vi "LV86_Histograph.vi"(3 "Image":T1 {"Dialogs" format="%.0b"}) -> (0 "Histogram":i32[](graph), 1 "Image Out":T1 {"Dialogs" format="%.0b"})   [LabVIEW 2024]
doc: "This VI automatically thresholds an image (clustering method). Pixels within the determined range maintain their original value, while pixels outside this range are given the value 0. (Does not work with color images)"
uses:
  <userlib>/ImageProcessing/QTLIB_2595_LV86/QT_Image.ctl
  <vilib>/Analysis/NI_AALPro.lvlib
panel:
  # "This VI automatically thresholds an image(clustering method).\nPixels within the determined range  maintain their original value, while pixels outside this range are given the value 0.   (Does not work with color images)"
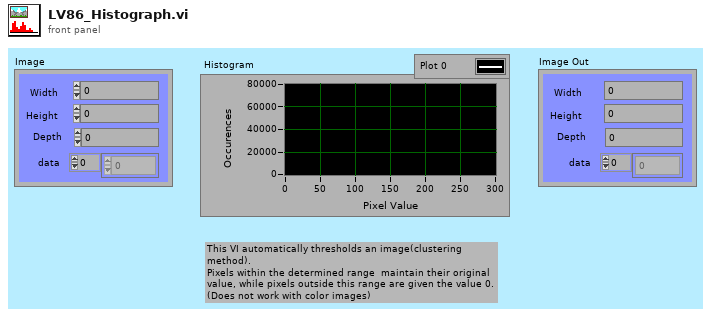
[diagram p1: front panel]
types:
  T1 = typedef "QT_Image.ctl" = cluster{"Width":i32, "Height":i32, "Depth":i32, "data":u8[], "Compressed data":u8[], "Color table":u32[], "Duration":i32, "Options":i32, "Timestamp":i32, "ID":i32, "Reserved":i32, "Dialogs":u32}
  T2 = cluster{i32, i32, "inclusion":enum32{"lower", "upper", "both", "neither"}}
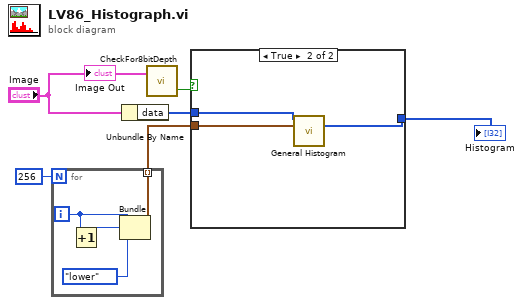
[diagram p0: block diagram]
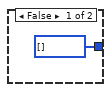
[diagram p2: hidden frame]
diagram:
  n1 = for {
    N: 256 -> [_]
    tunnel: [w7] -> w4 mode=indexing
    i -> [w9]
    n2 = Increment(x=w9) -> (x+1=w10:i32)
    n3 = Bundle(w9, w10, "inclusion"=enum32{"lower", "upper", "both", "neither"}."lower") -> (w7:T2)  [unwired: 1 out]
  }
  n4 = Unbundle By Name("Image") -> ("data"=w6:u8[])
  n5 = call <userlib>:"CheckFor8bitDepth.vi"("Image in"="Image") -> ("Success?"=w1:bool)  [unwired: 2 out]
  n6 = case shown="True" w1 {
    tunnel: w6 -> [_ w13]
    tunnel: w4 -> [_ w14]
    tunnel: [i32[] [] ("Histogram") w12] -> w3
    frame False {
    }
    frame True {
      n7 = call <vilib>:"General Histogram.vi"("X"=w13, "Bins"=w14) -> ("Histogram"=w12:i32[])  [unwired: 4 in, 9 out]
    }
  }
  "Histogram" <- w3
  "Image Out" <- "Image"
